vi "4155C Generate Logfile.vi"(0 "Ig":dbl format="%.2e", 1 "Id":dbl format="%.2e", 2 "Is":dbl format="%.2e", 3 "Drain":T2={"Drain Start"=0.0, "Drain Stop"=2.0, "Drain Compliance"=0.0001, "Drain Step"=1.0, "Drain PComp"=0.0, "Range mode"=0, "Range"=6} {"Range" max=11 scale=0.0..11.0; "Range mode" items=["Auto", "Limited", "Fixed"]; "Drain PComp" format="%^.2e"; "Drain Step" format="%^.4e"; "Drain Compliance" format="%^.2e"; "Drain Stop" format="%^.4e"; "Drain Start" format="%^.4e"}, 4 "Timings":T1={"integration time"=0, "Short/Long integration time"=0.00064, "hold time (sec)"=0.0, "delay time (sec)"=0.0, "Step Time (0 disables)"=0.0, "sweep method"=0, "Pulse period"=0.005, "Base voltage"=0.0, "Pulse width"=0.0005} {"Pulse width" min=0.0005 max=0.1 step=0.0001 format="%.4f"; "Base voltage" format="%^.4e"; "Pulse period" min=0.005 max=1.0 step=0.0001 format="%.4f"; "sweep method" items=["Continuous", "Pulsed"]; "Step Time (0 disables)" format="%.2f"; "delay time (sec)" format="%.4f"; "hold time (sec)" format="%.4f"; "Short/Long integration time" format="%^.0e"; "integration time" scale=0.0..2.0}, 5 "Gate":T3={"Gate Start"=0.0, "Gate Stop"=2.0, "Gate Step"=1.0, "Gate Compliance"=0.0001, "Gate PComp"=0.0, "Range mode"=0, "Range"=6} {"Range" max=11 scale=0.0..11.0; "Range mode" items=["Auto", "Limited", "Fixed"]; "Gate PComp" format="%.2e"; "Gate Compliance" format="%.2e"; "Gate Step" format="%.2f"; "Gate Stop" format="%.2f"; "Gate Start" format="%.2f"}, 6 "sweep mode":u16(ring)=1 items=["Single", "Double"], 7 "SMU4":cluster{"on/off":bool, "Voltage":dbl} {"Voltage" min=-100.0 max=100.0 format="%.2f"}, 8 "Output?":bool, 9 "Input I":dbl[](array[numeric]) format="%.2f", 10 "VG":dbl[](array[numeric]) format="%.2f", 11 "Path":path) -> ()   [LabVIEW 2016]
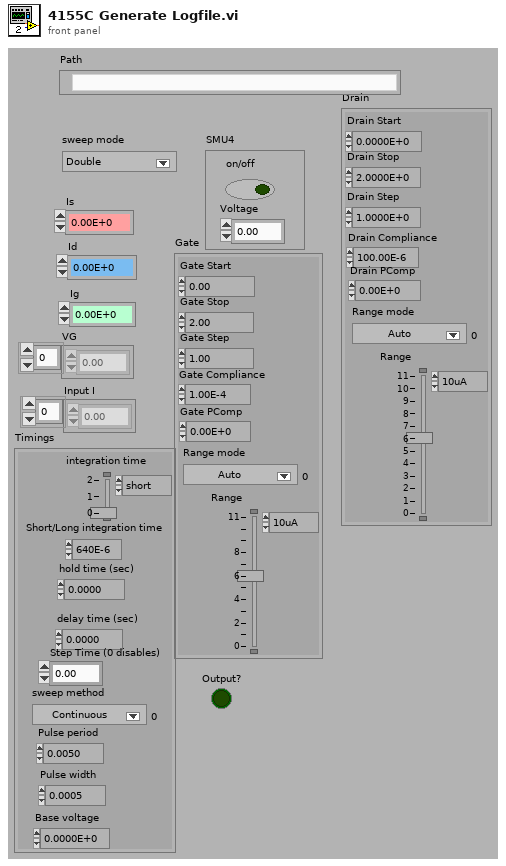
[diagram p1: front panel]
types:
  T1 = cluster{"integration time":u32, "Short/Long integration time":dbl, "hold time (sec)":dbl, "delay time (sec)":dbl, "Step Time (0 disables)":dbl, "sweep method":u16, "Pulse period":dbl, "Base voltage":dbl, "Pulse width":dbl}
  T2 = cluster{"Drain Start":dbl, "Drain Stop":dbl, "Drain Compliance":dbl, "Drain Step":dbl, "Drain PComp":dbl, "Range mode":u16, "Range":u8}
  T3 = cluster{"Gate Start":dbl, "Gate Stop":dbl, "Gate Step":dbl, "Gate Compliance":dbl, "Gate PComp":dbl, "Range mode":u16, "Range":u8}
  T4 = enum16{"open", "replace", "create", "open or create", "replace or create", "replace or create with confirmation"}
  T5 = enum16{"read/write", "read-only", "write-only", "write-only (truncate)"}
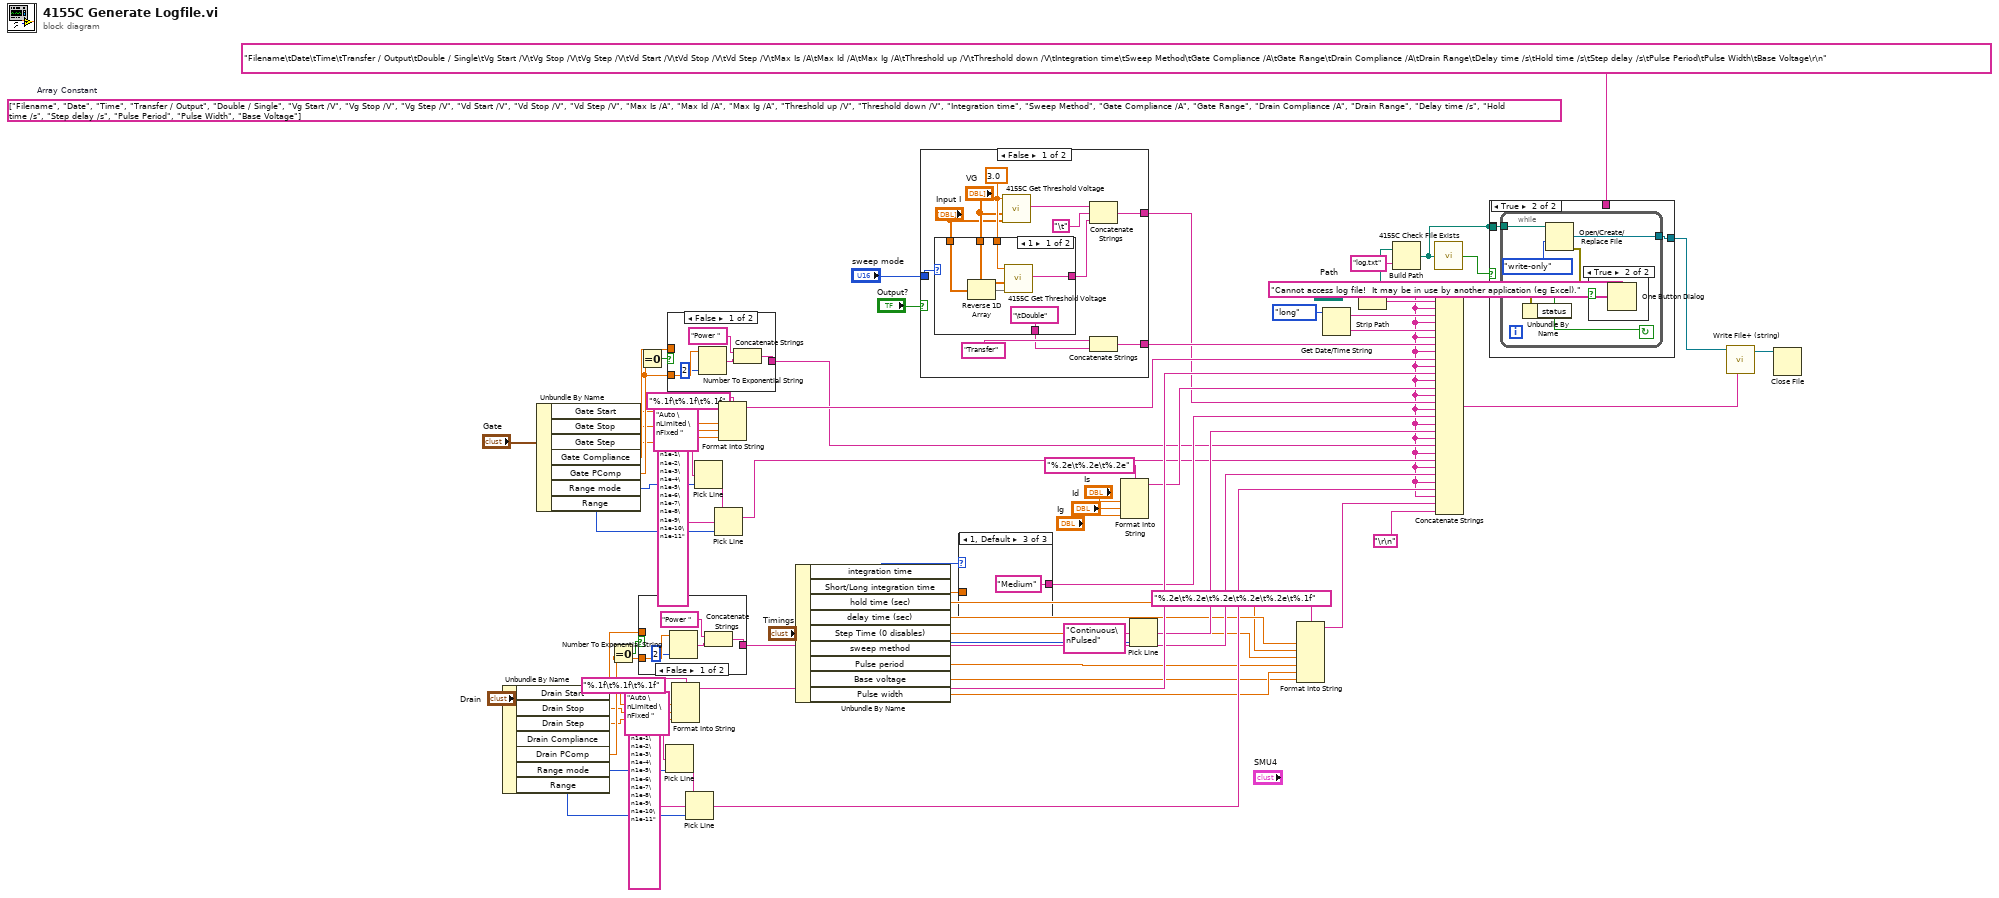
[diagram p0: block diagram]
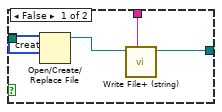
[diagram p2: hidden frame]
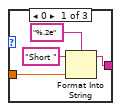
[diagram p4: hidden frame]
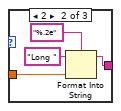
[diagram p5: hidden frame]
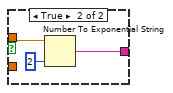
[diagram p6: hidden frame]
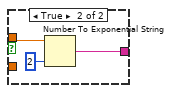
[diagram p7: hidden frame]
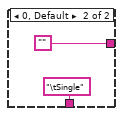
[diagram p8: hidden frame]
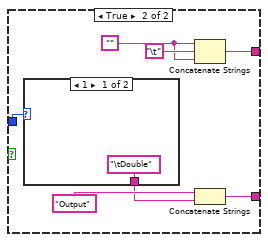
[diagram p9: hidden frame]
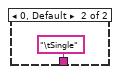
[diagram p10: hidden frame]
diagram:
  (unwired) string[] ["Filename", "Date", "Time", "Transfer / Output", "Double / Single", "Vg Start /V", "Vg Stop /V", "Vg Step /V", "Vd Start /V", "Vd Stop /V", "Vd Step /V", "Max Is /A", "Max Id /A", "Max Ig /A", "Threshold up /V", "Threshold down /V", "Integration time", "Sweep Method", "Gate Compliance /A", "Gate Range", "Drain Compliance /A", "Drain Range", "Delay time /s", "Hold time /s", "Step delay /s", "Pulse Period", "Pulse Width", "Base Voltage"]  # Array Constant
  w11 = "\t"
  n1 = Unbundle By Name("Drain") -> ("Drain Start"=w44:dbl, "Drain Stop"=w43:dbl, "Drain Step"=w42:dbl, "Drain Compliance"=w53:dbl, "Drain PComp"=w54:dbl, "Range mode"=w51:u16, "Range"=w52:u8)
  n2 = Unbundle By Name("Gate") -> ("Gate Start"=w49:dbl, "Gate Stop"=w48:dbl, "Gate Step"=w47:dbl, "Gate Compliance"=w61:dbl, "Gate PComp"=w59:dbl, "Range mode"=w62:u16, "Range"=w64:u8)
  n3 = Equal To 0?(x=w54) -> (x = 0?=w57:bool)
  n4 = Equal To 0?(x=w59) -> (x = 0?=w60:bool)
  n5 = case shown="False" w57 {
    tunnel: w53 -> [_ w79]
    tunnel: [w74 w78] -> w21
    tunnel: w54 -> [w76 _]
    frame False {
      n6 = Number To Exponential String(number=w76, precision (6)=i16 2) -> (E-format string=w75:string)  [unwired: 2 in]
      n7 = Concatenate Strings("Power " ("Substring"), w75) -> (w74:string)
    }
    frame True {
      n8 = Number To Exponential String(number=w79, precision (6)=i16 2) -> (E-format string=w78:string)  [unwired: 2 in]
    }
  }
  n9 = Pick Line(multi-line string="Auto \nLimited \nFixed ", line index=w51) -> (output string=w45:string)  [unwired: 1 in]
  n10 = case shown="False" w60 {
    tunnel: w61 -> [_ w87]
    tunnel: [w82 w86] -> w23
    tunnel: w59 -> [w84 _]
    frame False {
      n11 = Number To Exponential String(number=w84, precision (6)=i16 2) -> (E-format string=w83:string)  [unwired: 2 in]
      n12 = Concatenate Strings("Power " ("Substring"), w83) -> (w82:string)
    }
    frame True {
      n13 = Number To Exponential String(number=w87, precision (6)=i16 2) -> (E-format string=w86:string)  [unwired: 2 in]
    }
  }
  n14 = Format Into String(format string="%.1f\t%.1f\t%.1f" ("Format String"), w44, w43, w42) -> (resulting string=w34:string)  [unwired: 2 in, 1 out]
  n15 = Pick Line(string ("")=w45, multi-line string="1A\n1e-1\n1e-2\n1e-3\n1e-4\n1e-5\n1e-6\n1e-7\n1e-8\n1e-9\n1e-10\n1e-11", line index=w52) -> (output string=w20:string)
  n16 = Pick Line(multi-line string="Auto \nLimited \nFixed ", line index=w62) -> (output string=w63:string)  [unwired: 1 in]
  n17 = Pick Line(string ("")=w63, multi-line string="1A\n1e-1\n1e-2\n1e-3\n1e-4\n1e-5\n1e-6\n1e-7\n1e-8\n1e-9\n1e-10\n1e-11", line index=w64) -> (output string=w22:string)
  n18 = Format Into String(format string="%.1f\t%.1f\t%.1f" ("Format String"), w49, w48, w47) -> (resulting string=w35:string)  [unwired: 2 in, 1 out]
  n19 = Unbundle By Name("Timings") -> ("integration time"=w40:u32, "Short/Long integration time"=w39:dbl, "hold time (sec)"=w18:dbl, "delay time (sec)"=w19:dbl, "Step Time (0 disables)"=w17:dbl, "sweep method"=w25:u16, "Pulse period"=w16:dbl, "Base voltage"=w14:dbl, "Pulse width"=w15:dbl)
  n20 = case shown="False" "Output?" {
    tunnel: "sweep mode" -> [w95 w113]
    tunnel: [w89 w108] -> w28
    tunnel: [w88 w107] -> w36
    frame False {
      w98 = 3.0 ("Threshold ratio")
      n21 = case shown="1" w95 {
        tunnel: w98 -> [w104 _]
        tunnel: "VG" -> [w103 _]
        tunnel: "Input I" -> [w101 _]
        tunnel: [w100 ""] -> w92
        tunnel: ["\tDouble" "\tSingle"] -> w90
        frame 1 {
          n22 = Reverse 1D Array(array=w101) -> (reversed array=w102:dbl[])
          n23 = call "4155C Get Threshold Voltage.vi"("Input I"=w102, "VG"=w103, "Threshold ratio"=w104) -> ("Threshold Voltage"=w100:string)  [unwired: 8 in]
        }
        frame 0, Default {
        }
      }
      n24 = call "4155C Get Threshold Voltage.vi"("Input I"="Input I", "VG"="VG", "Threshold ratio"=w98) -> ("Threshold Voltage"=w94:string)  [unwired: 8 in]
      n25 = Concatenate Strings(w94, "\t", w92) -> (w89:string)
      n26 = Concatenate Strings("Transfer", w90) -> (w88:string)
    }
    frame True {
      w109 = ""
      n27 = case shown="1" w113 {
        tunnel: ["\tDouble" "\tSingle"] -> w110
        frame 1 {
        }
        frame 0, Default {
        }
      }
      n28 = Concatenate Strings(w109, "\t", w109) -> (w108:string)
      n29 = Concatenate Strings("Output", w110) -> (w107:string)
    }
  }
  n30 = case shown="1, Default" w40 {
    tunnel: w39 -> [w118 w122 _]
    tunnel: [w116 w120 "Medium"] -> w27
    frame 0 {
      n31 = Format Into String(format string="%.2e" ("Format String"), initial string="Short " ("Input String"), w118) -> (resulting string=w116:string)  [unwired: 1 in, 1 out]
    }
    frame 2 {
      n32 = Format Into String(format string="%.2e" ("Format String"), initial string="Long " ("Input String"), w122) -> (resulting string=w120:string)  [unwired: 1 in, 1 out]
    }
    frame 1, Default {
    }
  }
  n33 = Format Into String(format string="%.2e\t%.2e\t%.2e" ("Format String"), "Is", "Id", "Ig") -> (resulting string=w29:string)  [unwired: 2 in, 1 out]
  n34 = Pick Line(multi-line string="Continuous\nPulsed", line index=w25) -> (output string=w24:string)  [unwired: 1 in]
  n35 = Format Into String(format string="%.2e\t%.2e\t%.2e\t%.2e\t%.2e\t%.1f" ("Format String"), w19, w18, w17, w16, w15, w14) -> (resulting string=w12:string)  [unwired: 2 in, 1 out]
  n36 = Get Date/Time String(date format (0)=enum16{"short", "long", "abbreviated"}."long") -> (date string=w69:string, time string=w68:string)  [unwired: 2 in]
  n37 = Strip Path(path="Path") -> (stripped path=w8:path, name=w70:string)
  n38 = Build Path(base path=w8, name or relative path="log.txt") -> (appended path=w5:path)
  n39 = call "4155C Check File Exists.vi"("Path"=w5) -> ("Exists?"=w1:bool)
  n40 = Concatenate Strings(w70, w11, w69, w11, w68, w11, w36, w11, w35, w11, w34, w11, w29, w11, w28, w11, w27, w11, w24, w11, w23, w11, w22, w11, w21, w11, w20, w11, w12, "\r\n") -> (w4:string)
  n41 = case shown="True" w1 {
    tunnel: w5 -> [w129 w131]
    tunnel: "Filename\tDate\tTime\tTransfer / Output\tDouble / Single\tVg Start /V\tVg Stop /V\tVg Step /V\tVd Start /V\tVd Stop /V\tVd Step /V\tMax Is /A\tMax Id /A\tMax Ig /A\tThreshold up /V\tThreshold down /V\tIntegration time\tSweep Method\tGate Compliance /A\tGate Range\tDrain Compliance /A\tDrain Range\tDelay time /s\tHold time /s\tStep delay /s\tPulse Period\tPulse Width\tBase Voltage\r\n" ("format string") -> [w127 _]
    tunnel: [w126 w130] -> w3
    tunnel: w5 -> [_ _]
    frame False {
      n42 = Open/Create/Replace File(file path (use dialog)=w129, operation (0:open)=T4."create") -> (refnum out=w128:refnum<file>)  [unwired: 4 in, 2 out]
      n43 = call <vilib>:"Write File+ (string).vi"("string"=w127, "refnum"=w128) -> ("dup refnum"=w126:refnum<file>)  [unwired: 5 in, 2 out]
    }
    frame True {
      n44 = while {
        tunnel: [w135] -> w130
        tunnel: w131 -> [w136]
        stop <- w132 continue-if-true
        n45 = Open/Create/Replace File(file path (use dialog)=w136, access (0:read/write)=T5."write-only" ("open mode (0)")) -> (refnum out=w135:refnum<file>, error out=w133:errorcluster)  [unwired: 4 in, 1 out]
        n46 = Unbundle By Name(w133) -> ("status"=w132:bool)
        n47 = case shown="True" w132 {
          frame False {
          }
          frame True {
            n48 = One Button Dialog(message="Cannot access log file!  It may be in use by another application (eg Excel).") -> ()  [unwired: 1 in, 1 out]
          }
        }
      }
    }
  }
  n49 = call <vilib>:"Write File+ (string).vi"("string"=w4, "refnum"=w3) -> ("dup refnum"=w2:refnum<file>)  [unwired: 5 in, 2 out]
  n50 = Close File(refnum=w2) -> ()  [unwired: 1 in, 2 out]
